vi "Destroy.vi"(0 "reference in":refnum<class "SigMath.lvclass">, 5 "error in (no error)":errorcluster) -> (14 "reference out":refnum<class "SigMath.lvclass">, 19 "error out":errorcluster)   [LabVIEW 2020, in "SigMath.lvclass"]
doc: "Destructor."
uses:
  SigMath.lvclass
  API/Generic Utilities_class/Generic Utilities.lvclass
  API/GSwFormDSP_class/GSwFormDSP.lvclass
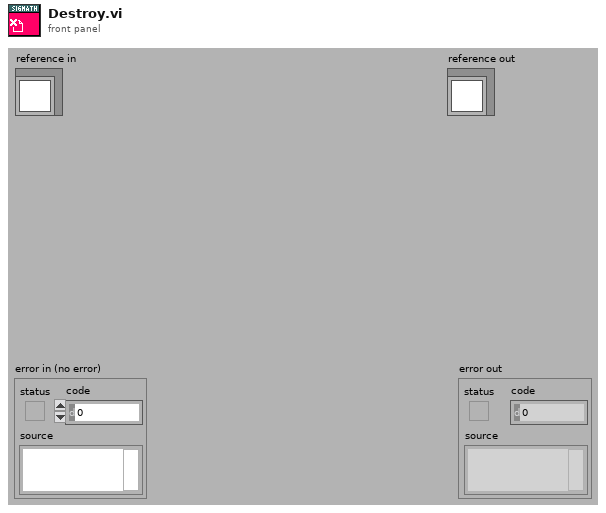
[diagram p1: front panel]
types:
  T1 = typedef "SigMath.lvclass/ObjectAttributes.ctl" = cluster{"SigMath Data":T2, "User CTRL Refs":T3}
  T2 = typedef "SigMath.lvclass/SigMath Data.ctl" = cluster{"New Time Data Obj?":bool, "GSwFormDSP":refnum<class "GSwFormDSP.lvclass">}
  T3 = typedef "SigMath.lvclass/SigMath User CTRL Refs.ctl" = cluster{"wForms":refnum<vi>, "Results wForms":refnum<vi>}
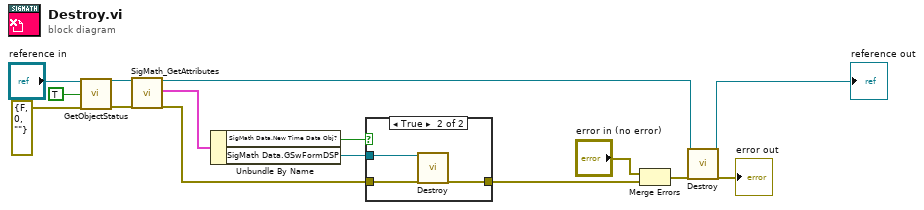
[diagram p0: block diagram]
diagram:
  n1 = call-dynamic "GetObjectStatus.vi"("reference in"="reference in", "simple info (F)"=TRUE ("simple info"), "error in (no error)"=errorcluster {"status"=FALSE, "code"=0, "source"=""}) -> ("reference out"=w9:refnum<class "SigMath.lvclass">, "error out"=w10:errorcluster)  [unwired: 5 in, 10 out]
  n2 = call "SigMath_GetAttributes.vi"("reference in"=w9, "error in (no error)"=w10) -> ("reference out"=w8:refnum<class "SigMath.lvclass">, "attributes"=w7:T1, "error out"=w2:errorcluster)  [unwired: 14 in, 1 out]
  n3 = Unbundle By Name(w7) -> ("SigMath Data.New Time Data Obj?"=w4:bool, "SigMath Data.GSwFormDSP"=w3:refnum<class "GSwFormDSP.lvclass">)
  n4 = case shown="True" w4 {
    tunnel: w3 -> [_ w19]
    tunnel: w2 -> [w16 w18]
    tunnel: [w16 w17] -> w1
    frame False {
    }
    frame True {
      n5 = call-dynamic "Destroy.vi"("reference in"=w19, "error in (no error)"=w18) -> ("error out"=w17:errorcluster)  [unwired: 16 in, 1 out]
    }
  }
  n6 = Merge Errors("error in (no error)", w1) -> (w14:errorcluster)
  n7 = call-parent "Destroy.vi"("reference in"=w8, "error in (no error)"=w14) -> ("reference out"=→"reference out":refnum<class "SigMath.lvclass">, "error out"=→"error out":errorcluster)  [unwired: 16 in]
